vi "AssignUnits.vi"(1 "Infuse Units":u16(ring)=1 items=["milliliters", "microliters", "nanoliters", "picoliters"], 2 "Numeric":dbl format="%#_13g") -> (0 "Numeric 2":dbl[unit])   [LabVIEW 2018]
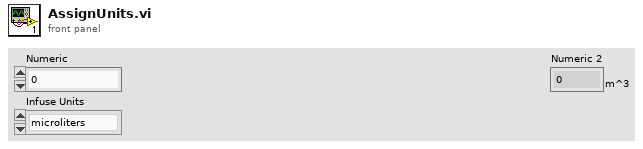
[diagram p1: front panel]
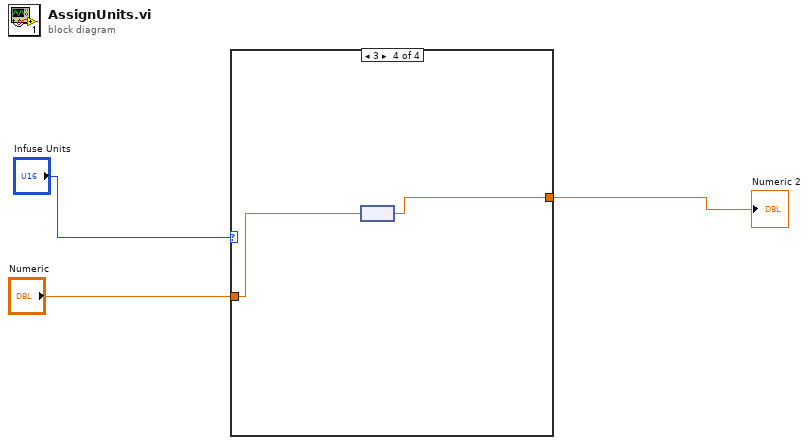
[diagram p0: block diagram]
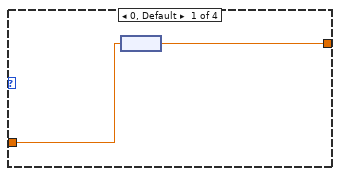
[diagram p2: hidden frame]
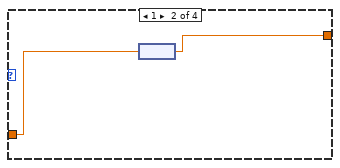
[diagram p3: hidden frame]
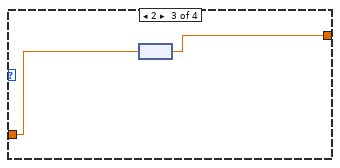
[diagram p4: hidden frame]
diagram:
  n1 = case shown="3" "Infuse Units" {
    tunnel: "Numeric" -> [w5 w6 w8 w10]
    tunnel: [w4 w7 w9 w11] -> w1
    frame 0, Default {
      n2 = node(w5) -> (w4:dbl[unit])
    }
    frame 1 {
      n3 = node(w6) -> (w7:dbl[unit])
    }
    frame 2 {
      n4 = node(w8) -> (w9:dbl[unit])
    }
    frame 3 {
      n5 = node(w10) -> (w11:dbl[unit])
    }
  }
  "Numeric 2" <- w1
